vi "Diagnostics.Channel.Engine.vi"(8 "error in":errorcluster, 11 "State Variables":T1={"TCP Refs"={"Connection List"=refnum, "listener ID"=refnum}, "Stop"=refnum, "Top VI"=refnum, "Parameters"={"Properties"={"Name"="", "CAN"={"CAN Interface"=enum."CAN0", "Baud Rate"=0, "Diagnostic Protocol"=enum."GMLAN", "Transport Protocol"=enum."ISO TP - Normal Mode", "Transmit ID"=0, "Receive ID"=0, "Transmit Extension"=0, "Receive Extension"=0, "Receive UUDT ID"=0, "Enable Stream"=TRUE, "VW TP Channel ID"=0, "Security"={"Source DLL Path"=path "", "Security Level"=1, "Target DLL Path"=path ""}, "Fill Frame"=FALSE, "Fill Byte"=255, "Termination"=FALSE}, "986x"={"Enable"=FALSE, "RIO Device"=0, "Bitfile"=path ""}, "Reads"=[], "Frames Lookup"=variant, "Writes"=[], "DPIDs"=[], "DPID Lookup"=variant, "DTC descriptor"={"DTC Byte Length"=2, "Status Byte Length"=1, "Add Data Byte Length"=1, "Byte Order"=enum."Motorola"}, "Created DTCs"=0}, "ChanRefs"={"ToVS.Reads"={"Name"="", "Write to VS Engine FIFO"=refnum, "Pairs"={"Refs"=[], "Values"=[]}}, "ToVS.DTCs"={"Name"="", "Write to VS Engine FIFO"=refnum, "Pairs"={"Refs"=[], "Values"=[]}}, "ToVS.DTCCount"={"Name"="", "Write to VS Engine FIFO"=refnum, "Pairs"={"Refs"=[], "Values"=[]}}, "ToVS.Status"={"Name"="", "Write to VS Engine FIFO"=refnum, "Pairs"={"Refs"=[], "Values"=[]}}, "FromVS.Writes"={"Name"="", "Read from VS Engine FIFO"=refnum, "Pairs"={"Refs"=[], "Values"=[]}}, "Cmds"={"Name"="", "Write to VS Engine FIFO"=refnum, "Read from VS Engine FIFO"=refnum, "Pairs"={"Chan Refs"=[], "Prev. Values"=[]}}, "Triggers"={"Name"="", "Write to VS Engine FIFO"=refnum, "Read from VS Engine FIFO"=refnum, "Pairs"={"Chan Refs"=[], "Prev. Values"=[]}}}}, "ADCS Connection"={"Diag CAN Handle"=0, "Transport Protocol"=enum."ISO TP - Normal Mode", "Receive Address Extension"=0, "Transmit Address Extension"=0, "Receive CAN Id"=0, "Transmit CAN Id"=0, "Diag CAN Queue"=refnum, "Log Frames ?"=FALSE, "My TP Address"=0, "Other TP Address"=0, "T1"=0, "T2"=0, "T3"=0, "T4"=0, "Tx SN"=0, "Block Size"=0, "Rx SN"=0, "VW TP Initialized?"=FALSE, "Tx block no"=0, "baud rate"=0, "Interface"="", "Channel Diag CAN Handle"=0, "UDP Connection ID"=refnum, "TCP Connection ID"=refnum, "Target IP Addr"=0, "Source Address"=0, "Target Address"=0, "Send Header NACK?"=FALSE, "DLL Handle"=0, "NAD"=0, "Time Stamp read first"=0.0, "Time Stamp read last"=0.0, "Time Stamp write first"=0.0, "Time Stamp write last"=0.0, "Time Stamp write"=0.0, "Time Stamp read"=0.0}, "XNET References"={"Database"="", "GMLAN DPID Session"="", "Cluster"=""}, "BufferedCmds"=refnum, "XNETEngine (GMLAN)"=refnum} {"Parameters"."ChanRefs"."Triggers"."Pairs"."Chan Refs" format="%.0x"; "Parameters"."ChanRefs"."Cmds"."Pairs"."Chan Refs" format="%.0x"; "Parameters"."ChanRefs"."ToVS.Status"."Pairs"."Refs" format="%.0x"; "Parameters"."ChanRefs"."ToVS.DTCCount"."Pairs"."Refs" format="%.0x"; "Parameters"."ChanRefs"."ToVS.DTCs"."Pairs"."Refs" format="%.0x"; "Parameters"."ChanRefs"."ToVS.Reads"."Pairs"."Refs" format="%.0x"; "Parameters"."Properties"."Writes"."Signals"."Byte Order" items=["Little Endian", "Big Endian"]; "Parameters"."Properties"."Writes"."Signals"."Data Type" items=["Signed", "Unsigned", "IEEE Float"]; "Parameters"."Properties"."CAN"."Fill Byte" format="%.0x"; "Parameters"."Properties"."CAN"."VW TP Channel ID" format="%.0x"; "Parameters"."Properties"."CAN"."Receive UUDT ID" format="%.0x"; "Parameters"."Properties"."CAN"."Receive Extension" format="%.0x"; "Parameters"."Properties"."CAN"."Transmit Extension" format="%.0x"; "Parameters"."Properties"."CAN"."Receive ID" format="%.0x"; "Parameters"."Properties"."CAN"."Transmit ID" format="%.0x"; "Parameters"."Properties"."Reads"."Signals"."Byte Order" items=["Little Endian", "Big Endian"]; "Parameters"."Properties"."Reads"."Signals"."Data Type" items=["Signed", "Unsigned", "IEEE Float"]}) -> (0 "error out":errorcluster)   [LabVIEW 2015, in "Diagnostics Addon Engine.lvlib"]
uses:
  Diagnostics Addon Engine.lvlib
  Types/Diagnostics.State.ctl
  Types/TCP.Refs.ctl
  STM/STM Lookup Table Ref.ctl
  Stop FG/Stop Global Ref.ctl
  Types/Engine.State.ctl
  Shared/Types/SysDef.Compile.Properties.ctl
  Shared/Types/CAN.ctl
  Shared/Types/CAN.Interface.ctl
  Shared/Types/Protocol.ctl
  Shared/Types/Transport.ctl
  Shared/Types/Security.ctl
  Shared/Types/986x.ctl
  Shared/Types/Frame.Compile.ctl
  Shared/Types/Type.ctl
  Shared/Types/Signal.ctl
  Shared/Types/DPID.ctl
  Shared/Types/DPID.Rate.ctl
  Shared/Types/DTCDescriptor.ctl
  Types/Engine.Refs.ctl
  Inline Async API/Controls/Write To VS Engine.ctl
  <vilib>/NI Veristand/Custom Device API/Data Reference.ctl
  Inline Async API/Controls/Read From VS Engine.ctl
  <vilib>/NI Veristand/Custom Device API/Block Data Reference.ctl
  Inline Async API/Controls/ReadWrite Data.ctl
  <vilib>/Automotive Diagnostic Command Set/Diagnostic Transport.llb/Diag Reference.ctl
  <vilib>/Automotive Diagnostic Command Set/Diagnostic Transport.llb/Transport Protocol Selector.ctl
  <vilib>/Automotive Diagnostic Command Set/Diagnostic Transport.llb/Diag CAN Frame Log.ctl
  Types/XNET.Refs.ctl
  <vilib>/NI/AMC/Message Queue.ctl
  <vilib>/NI/AMC/Message.ctl
  <vilib>/NI/Tools/Keyed Array/KeyedArray.ctl
  Stop FG/Stop Global Commands.ctl
  Shared/Types/Command.ctl
  Shared/Types/Command.Memory.ctl
  Shared/Types/Command.ReadDTC.ctl
  Shared/Types/Command.ReadDTCbyDTCNumber.ctl
  Shared/Types/Command.Communication.ctl
  Shared/Types/Command.IO.ctl
  GMLAN/_SubVIs/ReadFailureRecordData_readFailureRecordParameters_failureRecordIdentifier.ctl
  Shared/Types/Command.PassThru.Channel.ctl
  <vilib>/NI/AMC/Update Message Routing Info.vi
  <vilib>/NI/AMC/Create Multiple Messages.vi
  <vilib>/NI/AMC/Create Single Message.vi
  <vilib>/NI/AMC/Send Message.vi
  Error Handling API/Error Handling API.lvlib
  Stop FG/Stop FG.lvlib
  Shared/Diagnostics Addon Shared.lvlib
  <vilib>/NI/AMC/AMC.lvlib
  GMLAN/GMLAN.lvlib
  <vilib>/NI Veristand/Custom Device API/Custom Device API.lvlib
  <vilib>/NI/Tools/Keyed Array/Tools_KeyedArray.lvlib
  <vilib>/addons/Automotive Diagnostic Command Set/NI_Automotive Diagnostic Command Set.lvlib
  Inline Async API/Inline Async API.lvlib
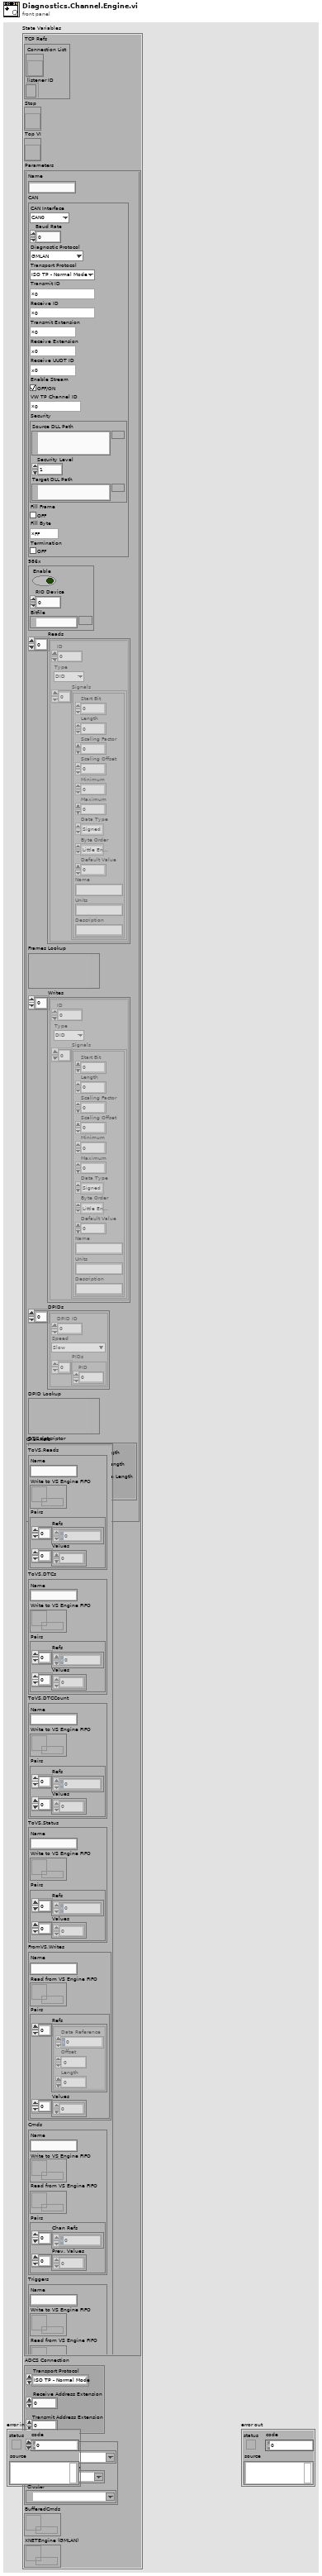
[diagram p1: front panel]
types:
  T1 = typedef "Diagnostics Addon Engine.lvlib/Diagnostics.State.ctl" = cluster{"TCP Refs":T2, "Stop":T4, "Top VI":refnum<vi>, "Parameters":T5, "ADCS Connection":T25, "XNET References":T27, "BufferedCmds":T28, "XNETEngine (GMLAN)":T28}
  T2 = typedef "Diagnostics Addon Engine.lvlib/TCP.Refs.ctl" = cluster{"Connection List":T3, "listener ID":refnum<k5>}
  T3 = typedef "Diagnostics Addon Engine.lvlib/STM Lookup Table Ref.ctl" = refnum<vi>
  T4 = typedef "Diagnostics Addon Engine.lvlib/Stop FG.lvlib/Stop Global Ref.ctl" = refnum<vi>
  T5 = typedef "Diagnostics Addon Engine.lvlib/Engine.State.ctl" = cluster{"Properties":T6, "ChanRefs":T19}
  T6 = typedef "Diagnostics Addon Shared.lvlib/SysDef.Compile.Properties.ctl" = cluster{"Name":string, "CAN":T7, "986x":T12, "Reads":T13[], "Frames Lookup":variant, "Writes":T13[], "DPIDs":T16[], "DPID Lookup":variant, "DTC descriptor":T18, "Created DTCs":u32}
  T7 = typedef "Diagnostics Addon Shared.lvlib/CAN.ctl" = cluster{"CAN Interface":T8, "Baud Rate":u32, "Diagnostic Protocol":T9, "Transport Protocol":T10, "Transmit ID":u32, "Receive ID":u32, "Transmit Extension":u8, "Receive Extension":u8, "Receive UUDT ID":u32, "Enable Stream":bool, "VW TP Channel ID":u32, "Security":T11, "Fill Frame":bool, "Fill Byte":u8, "Termination":bool}
  T8 = typedef "Diagnostics Addon Shared.lvlib/CAN.Interface.ctl" = enum16{"CAN0", "CAN1", "CAN2", "CAN3", "CAN4", "CAN5", "CAN6", "CAN7", "CAN8", "CAN9", "CAN10", "CAN11", "CAN12", "CAN13", "CAN14", "CAN15", "CAN16", "CAN17", "CAN18", "CAN19", "CAN20", "CAN21", "CAN22", "CAN23", "CAN24", "CAN25", "CAN26", "CAN27", "CAN28", "CAN29", "CAN30", "CAN31", "CAN32", "CAN33", "CAN34", "CAN35", "CAN36", "CAN37", "CAN38", "CAN39", "CAN40", "CAN41", "CAN42", "CAN43", "CAN44", "CAN45", "CAN46", "CAN47", "CAN48", "CAN49", "CAN50", "CAN51", "CAN52", "CAN53", "CAN54", "CAN55", "CAN56", "CAN57", "CAN58", "CAN59", "CAN60", "CAN61", "CAN62", "CAN63", "CAN 256 (Virtual)", "CAN 257 (Virtual)"}
  T9 = typedef "Diagnostics Addon Shared.lvlib/Protocol.ctl" = enum16{"GMLAN", "KWP-2000", "UDS", "User-Defined"}
  T10 = typedef "Diagnostics Addon Shared.lvlib/Transport.ctl" = enum16{"ISO TP - Normal Mode", "ISO TP - Mixed Mode", "VW TP 2.0", "Diagnostics on IP"}
  T11 = typedef "Diagnostics Addon Shared.lvlib/Security.ctl" = cluster{"Source DLL Path":path, "Security Level":u8, "Target DLL Path":path}
  T12 = typedef "Diagnostics Addon Shared.lvlib/986x.ctl" = cluster{"Enable":bool, "RIO Device":u16, "Bitfile":path}
  T13 = typedef "Diagnostics Addon Shared.lvlib/Frame.Compile.ctl" = cluster{"ID":u32, "Type":T14, "Signals":T15[]}
  T14 = typedef "Diagnostics Addon Shared.lvlib/Type.ctl" = enum16{"DID", "CDID", "PID", "CPID", "Read Memory", "Write Memory", "DTC Control", "IO Cmd", "IO Resp", "Routine Start Cmd", "Routine Start Resp", "Routine Request Cmd", "Routine Request Resp", "Routine Stop Cmd", "Routine Stop Resp", "UserDefined Cmd", "UserDefined Rsp"}
  T15 = typedef "Diagnostics Addon Shared.lvlib/Signal.ctl" = cluster{"Start Bit":u32, "Length":u32, "Scaling Factor":dbl, "Scaling Offset":dbl, "Minimum":dbl, "Maximum":dbl, "Data Type":u32, "Byte Order":u32, "Default Value":dbl, "Name":string, "Units":string, "Description":string}
  T16 = typedef "Diagnostics Addon Shared.lvlib/DPID.ctl" = cluster{"DPID ID":u8, "Speed":T17, "PIDs":u16[]}
  T17 = typedef "Diagnostics Addon Shared.lvlib/DPID.Rate.ctl" = enum16{"Slow", "Medium", "Fast"}
  T18 = typedef "Diagnostics Addon Shared.lvlib/DTCDescriptor.ctl" = cluster{"DTC Byte Length":i32, "Status Byte Length":i32, "Add Data Byte Length":i32, "Byte Order":enum16{"Motorola", "Intel"}}
  T19 = typedef "Diagnostics Addon Engine.lvlib/Engine.Refs.ctl" = cluster{"ToVS.Reads":T20, "ToVS.DTCs":T20, "ToVS.DTCCount":T20, "ToVS.Status":T20, "FromVS.Writes":T22, "Cmds":T24, "Triggers":T24}
  T20 = typedef "Diagnostics Addon Engine.lvlib/Inline Async API.lvlib/Write To VS Engine.ctl" = cluster{"Name":string, "Write to VS Engine FIFO":refnum<k33>, "Pairs":cluster{"Refs":T21[], "Values":dbl[]}}
  T21 = typedef "Custom Device API.lvlib/Data Reference.ctl" = i32
  T22 = typedef "Diagnostics Addon Engine.lvlib/Inline Async API.lvlib/Read From VS Engine.ctl" = cluster{"Name":string, "Read from VS Engine FIFO":refnum<k33>, "Pairs":cluster{"Refs":T23[], "Values":dbl[]}}
  T23 = typedef "Custom Device API.lvlib/Block Data Reference.ctl" = cluster{"Data Reference":T21, "Offset":u64, "Length":u64}
  T24 = typedef "Diagnostics Addon Engine.lvlib/Inline Async API.lvlib/ReadWrite Data.ctl" = cluster{"Name":string, "Write to VS Engine FIFO":refnum<k33>, "Read from VS Engine FIFO":refnum<k33>, "Pairs":cluster{"Chan Refs":T21[], "Prev. Values":dbl[]}}
  T25 = typedef "NI_Automotive Diagnostic Command Set.lvlib/Diag Reference.ctl" = cluster{"Diag CAN Handle":u32, "Transport Protocol":T26, "Receive Address Extension":u8, "Transmit Address Extension":u8, "Receive CAN Id":u32, "Transmit CAN Id":u32, "Diag CAN Queue":refnum<queue>, "Log Frames ?":bool, "My TP Address":u8, "Other TP Address":u8, "T1":u16, "T2":u16, "T3":u16, "T4":u16, "Tx SN":u8, "Block Size":u8, "Rx SN":u8, "VW TP Initialized?":bool, "Tx block no":u8, "baud rate":u32, "Interface":string, "Channel Diag CAN Handle":u32, "UDP Connection ID":refnum<k16>, "TCP Connection ID":refnum<k5>, "Target IP Addr":u32, "Source Address":u16, "Target Address":u16, "Send Header NACK?":bool, "DLL Handle":u32, "NAD":u8, "Time Stamp read first":dbl, "Time Stamp read last":dbl, "Time Stamp write first":dbl, "Time Stamp write last":dbl, "Time Stamp write":dbl, "Time Stamp read":dbl}
  T26 = typedef "NI_Automotive Diagnostic Command Set.lvlib/Transport Protocol Selector.ctl" = enum16{"ISO TP - Normal Mode", "ISO TP - Mixed Mode", "VW TP 2.0", "Diagnostics on IP", "ISO TP LIN"}
  T27 = typedef "Diagnostics Addon Engine.lvlib/XNET.Refs.ctl" = cluster{"Database":refnum<k21>, "GMLAN DPID Session":refnum<k21>, "Cluster":refnum<k21>}
  T28 = typedef "AMC.lvlib/Message Queue.ctl" = refnum<queue>
  T29 = typedef "Diagnostics Addon Engine.lvlib/Stop FG.lvlib/Stop Global Commands.ctl" = enum16{"Write", "Read", "Reset"}
  T30 = typedef "Diagnostics Addon Shared.lvlib/Command.ctl" = enum8{"None", "EnableDiagnosticSession", "DisableDiagnosticSession", "ReadDataIdentifiers", "ReadDataIdentifier", "WriteDataIndentifier", "ReadPIDsOnDemand", "ReadPIDOnDemand", "WriteCPID", "WriteMemory", "ReadMemory", "ReadDTCs", "ClearDTCs", "ControlDTC", "ForceTesterPresent", "DisableNormalCommunication", "ReturnToNormalMode", "InputOutputControl", "StartRoutine", "RequestRoutineStatus", "StopRoutine", "ECUReset", "UnlockECU", "ClearSuccessBit", "ConfigureandStartPIDs", "StopPIDs", "StartDTCs", "EnableChangeDTCCount", "DisableChangeDTCCount", "ReadFailureRecordParameters", "PassThru Channel Based", "EnableRepeatingTesterPresent", "DisableRepeatingTesterPresent"}
  T31 = typedef "Diagnostics Addon Shared.lvlib/Command.Memory.ctl" = cluster{"Address":u64, "Service Type":u32, "Address Length":u8, "Size Length":u8}
  T32 = typedef "Diagnostics Addon Shared.lvlib/Command.ReadDTC.ctl" = cluster{"Extension":u32, "Mask":u32, "Mode":u32}
  T33 = typedef "Diagnostics Addon Shared.lvlib/Command.ReadDTCbyDTCNumber.ctl" = cluster{"DTC":u16, "FailTypeByte":u8}
  T34 = typedef "Diagnostics Addon Shared.lvlib/Command.Communication.ctl" = cluster{"Type":u8, "CommType":u8}
  T35 = typedef "Diagnostics Addon Shared.lvlib/Command.IO.ctl" = cluster{"ID":u16, "Mode":u8}
  T36 = typedef "GMLAN.lvlib/ReadFailureRecordData_readFailureRecordParameters_failureRecordIdentifier.ctl" = cluster{"failureRecordNumber":u8, "DTC ID":u16, "DTCFailureType":u8}
  T37 = typedef "Diagnostics Addon Shared.lvlib/Command.PassThru.Channel.ctl" = cluster{"Service":u64, "Service Length":u8, "Data Length":u32, "Response Required":bool}
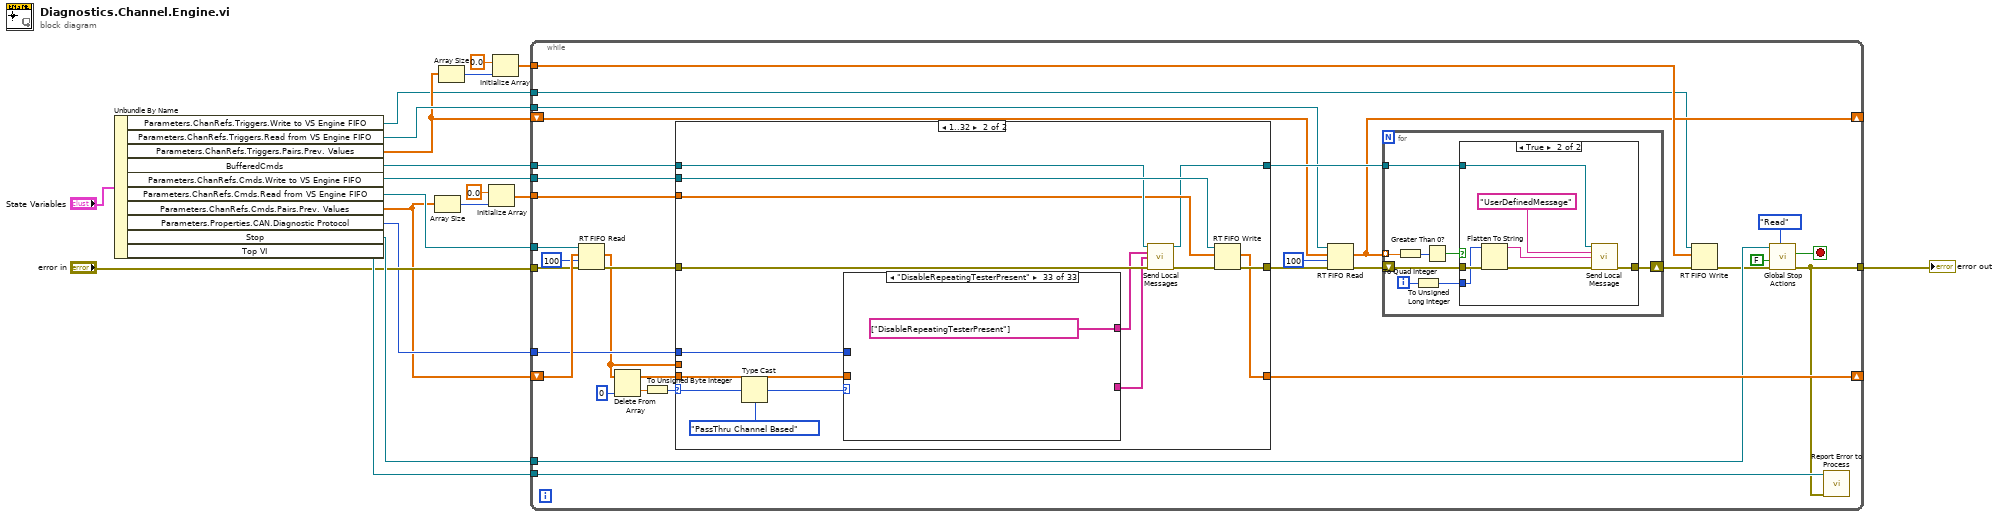
[diagram p0: block diagram]
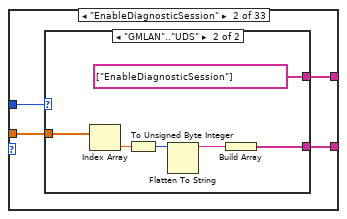
[diagram p5: hidden frame]
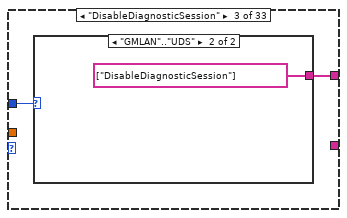
[diagram p7: hidden frame]
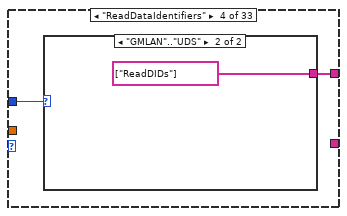
[diagram p9: hidden frame]
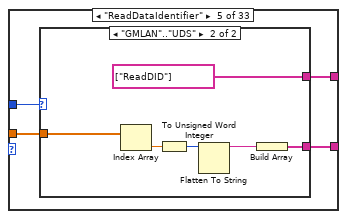
[diagram p11: hidden frame]
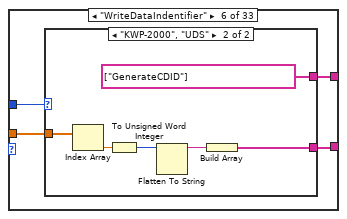
[diagram p13: hidden frame]
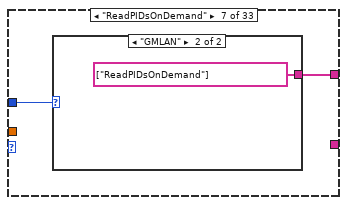
[diagram p15: hidden frame]
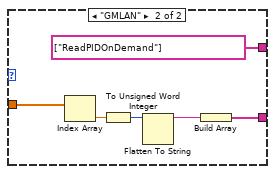
[diagram p18: hidden frame]
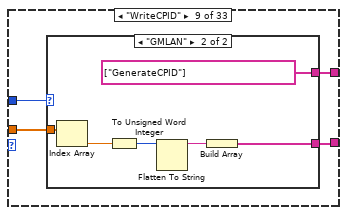
[diagram p19: hidden frame]
diagram:
  n1 = Unbundle By Name("State Variables") -> ("Parameters.ChanRefs.Triggers.Write to VS Engine FIFO"=w1:refnum<k33>, "Parameters.ChanRefs.Triggers.Read from VS Engine FIFO"=w3:refnum<k33>, "Parameters.ChanRefs.Triggers.Pairs.Prev. Values"=w2:dbl[], "BufferedCmds"=w12:T28, "Parameters.ChanRefs.Cmds.Write to VS Engine FIFO"=w13:refnum<k33>, "Parameters.ChanRefs.Cmds.Read from VS Engine FIFO"=w14:refnum<k33>, "Parameters.ChanRefs.Cmds.Pairs.Prev. Values"=w8:dbl[], "Parameters.Properties.CAN.Diagnostic Protocol"=w11:T9, "Stop"=w18:T4, "Top VI"=w17:refnum<vi>)
  n2 = Array Size(array=w8) -> (size(s)=w9:i32)
  n3 = Array Size(array=w2) -> (size(s)=w6:i32)
  n4 = Initialize Array(0.0 ("element"), w9) -> (w7:dbl[])
  n5 = Initialize Array(0.0 ("element"), w6) -> (w4:dbl[])
  n6 = while {
    tunnel: w14 -> [w46]
    shift-right: [w44] -> _
    shift-left: w8 -> [w45]
    tunnel: w18 -> [w40]
    tunnel: w17 -> [w39]
    tunnel: [w38] -> w16
    tunnel: "error in" -> [w36]
    tunnel: w13 -> [w35]
    tunnel: w12 -> [w34]
    tunnel: w11 -> [w33]
    tunnel: w7 -> [w30]
    tunnel: w4 -> [w25]
    tunnel: w3 -> [w23]
    shift-right: [w21] -> _
    shift-left: w2 -> [w22]
    tunnel: w1 -> [w20]
    stop <- w37 stop-if-true
    n7 = RT FIFO Read(0:w46, 1:w45, 2:100 ("timeout in ms (0)"), 3:w36) -> (9:w29:dbl[], 11:w51:errorcluster)  [unwired: 3 out]
    n8 = Delete From Array(array=w29, index=0) -> (deleted portion=w49:dbl, array with subset deleted=w47:dbl[])  [unwired: 1 in]
    n9 = To Unsigned Byte Integer(number=w49) -> (unsigned 8bit integer=w48:u8)
    n10 = case shown="1..32" w48 {
      selector: w48 -> [_ w73]
      tunnel: w51 -> [w70 w83]
      tunnel: w47 -> [_ w81]
      tunnel: [w69 w72] -> w44
      tunnel: [w70 w84] -> w31
      tunnel: w35 -> [_ w78]
      tunnel: w34 -> [w68 w75]
      tunnel: w33 -> [_ w74]
      tunnel: w30 -> [_ w72]
      tunnel: w29 -> [w69 _]
      tunnel: [w68 w71] -> w24
      frame 0, Default {
      }
      frame 1..32 {
        n11 = Type Cast(type=Command."PassThru Channel Based", x=w73) -> (*(type *) &x=w77:T30)
        n12 = case shown="\"DisableRepeatingTesterPresent\"" w77 {
          tunnel: w81 -> [_ w87 _ _ w103 w113 _ w126 w136 w145 w159 w174 w198 w208 w218 w229 _ w245 w259 w269 w279 w290 _ _ _ _ w310 w320 _ w336 w361 _ _]
          tunnel: [_ w88 w96 w99 w104 w114 w122 w127 w137 w147 w161 w175 w199 w209 w219 w230 w242 w247 w261 w271 w281 w291 w299 string[] ["ClearSuccessBit"] w303 w306 w311 w321 w330 w338 string[] ["ChannelPassThru"] string[] ["EnableRepeatingTesterPresent"] string[] ["DisableRepeatingTesterPresent"]] -> w80
          tunnel: [_ w86 _ _ w102 w112 _ w125 w135 w144 w158 w173 w197 w207 w217 w228 _ w244 w258 w268 w278 w289 _ _ _ _ w309 w319 w329 w337 w360 _ _] -> w79
          tunnel: w74 -> [_ w85 w95 w98 w101 w111 w121 w124 w134 w146 w160 w172 w196 w206 w216 w227 w241 w246 w260 w270 w280 w288 w298 _ w302 w305 w308 w318 w328 w335 _ _ _]
          frame "None" {
          }
          frame "EnableDiagnosticSession" {
            n13 = case shown="\"GMLAN\"..\"UDS\"" w85 {
              tunnel: [_ string[] ["EnableDiagnosticSession"]] -> w88
              tunnel: w87 -> [_ w90]
              tunnel: [_ w89] -> w86
              frame "User-Defined" {
              }
              frame "GMLAN".."UDS" {
                n14 = Index Array(array=w90) -> (element=w93:dbl)  [unwired: 1 in]
                n15 = To Unsigned Byte Integer(number=w93) -> (unsigned 8bit integer=w92:u8)
                n16 = Flatten To String(anything=w92) -> (data string=w91:string)  [unwired: 3 in, 2 out]
                n17 = Build Array(w91) -> (w89:string[])
              }
            }
          }
          frame "DisableDiagnosticSession" {
            n18 = case shown="\"GMLAN\"..\"UDS\"" w95 {
              tunnel: [_ string[] ["DisableDiagnosticSession"]] -> w96
              frame "User-Defined" {
              }
              frame "GMLAN".."UDS" {
              }
            }
          }
          frame "ReadDataIdentifiers" {
            n19 = case shown="\"GMLAN\"..\"UDS\"" w98 {
              tunnel: [_ string[] ["ReadDIDs"]] -> w99
              frame "User-Defined" {
              }
              frame "GMLAN".."UDS" {
              }
            }
          }
          frame "ReadDataIdentifier" {
            n20 = case shown="\"GMLAN\"..\"UDS\"" w101 {
              tunnel: [_ string[] ["ReadDID"]] -> w104
              tunnel: w103 -> [_ w106]
              tunnel: [_ w105] -> w102
              frame "User-Defined" {
              }
              frame "GMLAN".."UDS" {
                n21 = Index Array(array=w106) -> (element=w109:dbl)  [unwired: 1 in]
                n22 = To Unsigned Word Integer(number=w109) -> (unsigned 16bit integer=w108:u16)
                n23 = Flatten To String(anything=w108) -> (data string=w107:string)  [unwired: 3 in, 2 out]
                n24 = Build Array(w107) -> (w105:string[])
              }
            }
          }
          frame "WriteDataIndentifier" {
            n25 = case shown="\"KWP-2000\", \"UDS\"" w111 {
              tunnel: [_ string[] ["GenerateCDID"]] -> w114
              tunnel: w113 -> [_ w119]
              tunnel: [_ w118] -> w112
              frame "GMLAN", "User-Defined" {
              }
              frame "KWP-2000", "UDS" {
                n26 = Index Array(array=w119) -> (element=w117:dbl)  [unwired: 1 in]
                n27 = To Unsigned Word Integer(number=w117) -> (unsigned 16bit integer=w115:u16)
                n28 = Flatten To String(anything=w115) -> (data string=w116:string)  [unwired: 3 in, 2 out]
                n29 = Build Array(w116) -> (w118:string[])
              }
            }
          }
          frame "ReadPIDsOnDemand" {
            n30 = case shown="\"GMLAN\"" w121 {
              tunnel: [_ string[] ["ReadPIDsOnDemand"]] -> w122
              frame Default {
              }
              frame "GMLAN" {
              }
            }
          }
          frame "ReadPIDOnDemand" {
            n31 = case shown="Default" w124 {
              tunnel: [_ string[] ["ReadPIDOnDemand"]] -> w127
              tunnel: w126 -> [_ w129]
              tunnel: [_ w128] -> w125
              frame Default {
              }
              frame "GMLAN" {
                n32 = Index Array(array=w129) -> (element=w132:dbl)  [unwired: 1 in]
                n33 = To Unsigned Word Integer(number=w132) -> (unsigned 16bit integer=w131:u16)
                n34 = Flatten To String(anything=w131) -> (data string=w130:string)  [unwired: 3 in, 2 out]
                n35 = Build Array(w130) -> (w128:string[])
              }
            }
          }
          frame "WriteCPID" {
            n36 = case shown="\"GMLAN\"" w134 {
              tunnel: [_ string[] ["GenerateCPID"]] -> w137
              tunnel: w136 -> [_ w142]
              tunnel: [_ w141] -> w135
              frame Default {
              }
              frame "GMLAN" {
                n37 = Index Array(array=w142) -> (element=w140:dbl)  [unwired: 1 in]
                n38 = To Unsigned Word Integer(number=w140) -> (unsigned 16bit integer=w138:u16)
                n39 = Flatten To String(anything=w138) -> (data string=w139:string)  [unwired: 3 in, 2 out]
                n40 = Build Array(w139) -> (w141:string[])
              }
            }
          }
          frame "WriteMemory" {
            n41 = case shown="\"KWP-2000\", \"UDS\"" w146 {
              tunnel: [_ string[] ["WriteMemory"]] -> w147
              tunnel: w145 -> [_ w149]
              tunnel: [_ w156] -> w144
              frame "GMLAN", "User-Defined" {
              }
              frame "KWP-2000", "UDS" {
                n42 = Index Array(array=w149) -> (element #1=w153:dbl, element #2=w154:dbl, element #3=w152:dbl, element #4=w151:dbl)  [unwired: 4 in]
                n43 = Bundle By Name(cluster=T31 {"Address"=0, "Service Type"=0, "Address Length"=0, "Size Length"=0}, "Address"=w153, "Service Type"=w154, "Address Length"=w152, "Size Length"=w151) -> (w155:T31)
                n44 = Flatten To String(anything=w155) -> (data string=w150:string)  [unwired: 3 in, 2 out]
                n45 = Build Array(w150) -> (w156:string[])
              }
            }
          }
          frame "ReadMemory" {
            n46 = case shown="\"GMLAN\", \"User-Defined\"" w160 {
              tunnel: [_ string[] ["ReadMemory"]] -> w161
              tunnel: w159 -> [_ w170]
              tunnel: [_ w168] -> w158
              frame "GMLAN", "User-Defined" {
              }
              frame "KWP-2000", "UDS" {
                n47 = Index Array(array=w170) -> (element #1=w164:dbl, element #2=w165:dbl, element #3=w163:dbl, element #4=w162:dbl)  [unwired: 4 in]
                n48 = Bundle By Name(cluster=T31 {"Address"=0, "Service Type"=0, "Address Length"=0, "Size Length"=0}, "Address"=w164, "Service Type"=w165, "Address Length"=w163, "Size Length"=w162) -> (w166:T31)
                n49 = Flatten To String(anything=w166) -> (data string=w169:string)  [unwired: 3 in, 2 out]
                n50 = Build Array(w169) -> (w168:string[])
              }
            }
          }
          frame "ReadDTCs" {
            n51 = case shown="\"User-Defined\"" w172 {
              tunnel: [string[] ["ReadDTCs"] _ string[] ["ReadDTCByDTCNumber"]] -> w175
              tunnel: w174 -> [w183 _ w192]
              tunnel: [w181 _ w191] -> w173
              frame "KWP-2000", "UDS" {
                n52 = To Unsigned Long Integer(number=w183) -> (unsigned 32bit integer=w185:u32[])
                n53 = Index Array(array=w185) -> (element #1=w177:u32, element #2=w178:u32, element #3=w179:u32)  [unwired: 3 in]
                n54 = Bundle By Name(cluster=T32 {"Extension"=0, "Mask"=0, "Mode"=0}, "Extension"=w177, "Mask"=w178, "Mode"=w179) -> (w176:T32)
                n55 = Flatten To String(anything=w176) -> (data string=w184:string)  [unwired: 3 in, 2 out]
                n56 = Build Array(w184) -> (w181:string[])
              }
              frame "User-Defined" {
              }
              frame "GMLAN" {
                n57 = Index Array(array=w192) -> (element #1=w194:dbl, element #2=w190:dbl)  [unwired: 2 in]
                n58 = To Unsigned Word Integer(number=w194) -> (unsigned 16bit integer=w187:u16)
                n59 = To Unsigned Byte Integer(number=w190) -> (unsigned 8bit integer=w189:u8)
                n60 = Bundle By Name(cluster=T33 {"DTC"=0, "FailTypeByte"=0}, "DTC"=w187, "FailTypeByte"=w189) -> (w186:T33)
                n61 = Flatten To String(anything=w186) -> (data string=w193:string)  [unwired: 3 in, 2 out]
                n62 = Build Array(w193) -> (w191:string[])
              }
            }
          }
          frame "ClearDTCs" {
            n63 = case shown="\"User-Defined\"" w196 {
              tunnel: [_ string[] ["ClearDTCs"]] -> w199
              tunnel: w198 -> [_ w201]
              tunnel: [_ w200] -> w197
              frame "User-Defined" {
              }
              frame "GMLAN".."UDS" {
                n64 = Index Array(array=w201) -> (element=w204:dbl)  [unwired: 1 in]
                n65 = To Unsigned Long Integer(number=w204) -> (unsigned 32bit integer=w203:u32)
                n66 = Flatten To String(anything=w203) -> (data string=w202:string)  [unwired: 3 in, 2 out]
                n67 = Build Array(w202) -> (w200:string[])
              }
            }
          }
          frame "ControlDTC" {
            n68 = case shown="\"KWP-2000\", \"UDS\"" w206 {
              tunnel: [_ string[] ["ControlDTC"]] -> w209
              tunnel: w208 -> [_ w211]
              tunnel: [_ w210] -> w207
              frame "GMLAN", "User-Defined" {
              }
              frame "KWP-2000", "UDS" {
                n69 = Index Array(array=w211) -> (element=w214:dbl)  [unwired: 1 in]
                n70 = To Unsigned Long Integer(number=w214) -> (unsigned 32bit integer=w213:u32)
                n71 = Flatten To String(anything=w213) -> (data string=w212:string)  [unwired: 3 in, 2 out]
                n72 = Build Array(w212) -> (w210:string[])
              }
            }
          }
          frame "ForceTesterPresent" {
            n73 = case shown="\"User-Defined\"" w216 {
              tunnel: [_ string[] ["ForceTesterPresent"]] -> w219
              tunnel: w218 -> [_ w225]
              tunnel: [_ w224] -> w217
              frame "User-Defined" {
              }
              frame "GMLAN".."UDS" {
                n74 = Index Array(array=w225) -> (element=w223:dbl)  [unwired: 1 in]
                n75 = To Unsigned Byte Integer(number=w223) -> (unsigned 8bit integer=w220:u8)
                n76 = Number To Boolean Array(number=w220) -> (Boolean array=w221:bool[])
                n77 = Flatten To String(anything=w221) -> (data string=w222:string)  [unwired: 3 in, 2 out]
                n78 = Build Array(w222) -> (w224:string[])
              }
            }
          }
          frame "DisableNormalCommunication" {
            n79 = case shown="\"User-Defined\"" w227 {
              tunnel: [_ string[] ["DisableNormalCommunication"]] -> w230
              tunnel: w229 -> [_ w232]
              tunnel: [_ w231] -> w228
              frame "User-Defined" {
              }
              frame "GMLAN".."UDS" {
                n80 = Index Array(array=w232) -> (element #1=w237:dbl, element #2=w238:dbl)  [unwired: 2 in]
                n81 = To Unsigned Byte Integer(number=w238) -> (unsigned 8bit integer=w235:u8)
                n82 = To Unsigned Byte Integer(number=w237) -> (unsigned 8bit integer=w236:u8)
                n83 = Bundle By Name(cluster=T34 {"Type"=0, "CommType"=0} ("Cluster"), "Type"=w236, "CommType"=w235) -> (w234:T34)
                n84 = Flatten To String(anything=w234) -> (data string=w239:string)  [unwired: 3 in, 2 out]
                n85 = Build Array(w239) -> (w231:string[])
              }
            }
          }
          frame "ReturnToNormalMode" {
            n86 = case shown="\"User-Defined\"" w241 {
              tunnel: [_ string[] ["ReturnToNormalMode"]] -> w242
              frame "User-Defined" {
              }
              frame "GMLAN".."UDS" {
              }
            }
          }
          frame "InputOutputControl" {
            n87 = case shown="\"KWP-2000\", \"UDS\"" w246 {
              tunnel: [_ string[] ["InputOutputControl"]] -> w247
              tunnel: w245 -> [_ w255]
              tunnel: [_ w248] -> w244
              frame "GMLAN", "User-Defined" {
              }
              frame "KWP-2000", "UDS" {
                n88 = Index Array(array=w255) -> (element #1=w253:dbl, element #2=w254:dbl)  [unwired: 2 in]
                n89 = To Unsigned Byte Integer(number=w254) -> (unsigned 8bit integer=w250:u8)
                n90 = To Unsigned Word Integer(number=w253) -> (unsigned 16bit integer=w251:u16)
                n91 = Bundle By Name(cluster=T35 {"ID"=0, "Mode"=0}, "ID"=w251, "Mode"=w250) -> (w249:T35)
                n92 = Flatten To String(anything=w249) -> (data string=w256:string)  [unwired: 3 in, 2 out]
                n93 = Build Array(w256) -> (w248:string[])
              }
            }
          }
          frame "StartRoutine" {
            n94 = case shown="\"KWP-2000\", \"UDS\"" w260 {
              tunnel: [_ string[] ["StartRoutine"]] -> w261
              tunnel: w259 -> [_ w266]
              tunnel: [_ w262] -> w258
              frame "GMLAN", "User-Defined" {
              }
              frame "KWP-2000", "UDS" {
                n95 = Index Array(array=w266) -> (element=w265:dbl)  [unwired: 1 in]
                n96 = To Unsigned Word Integer(number=w265) -> (unsigned 16bit integer=w263:u16)
                n97 = Flatten To String(anything=w263) -> (data string=w264:string)  [unwired: 3 in, 2 out]
                n98 = Build Array(w264) -> (w262:string[])
              }
            }
          }
          frame "RequestRoutineStatus" {
            n99 = case shown="\"KWP-2000\", \"UDS\"" w270 {
              tunnel: [_ string[] ["RequestRoutineStatus"]] -> w271
              tunnel: w269 -> [_ w273]
              tunnel: [_ w272] -> w268
              frame "GMLAN", "User-Defined" {
              }
              frame "KWP-2000", "UDS" {
                n100 = Index Array(array=w273) -> (element=w276:dbl)  [unwired: 1 in]
                n101 = To Unsigned Word Integer(number=w276) -> (unsigned 16bit integer=w274:u16)
                n102 = Flatten To String(anything=w274) -> (data string=w275:string)  [unwired: 3 in, 2 out]
                n103 = Build Array(w275) -> (w272:string[])
              }
            }
          }
          frame "StopRoutine" {
            n104 = case shown="\"KWP-2000\", \"UDS\"" w280 {
              tunnel: [_ string[] ["StopRoutine"]] -> w281
              tunnel: w279 -> [_ w283]
              tunnel: [_ w282] -> w278
              frame "GMLAN", "User-Defined" {
              }
              frame "KWP-2000", "UDS" {
                n105 = Index Array(array=w283) -> (element=w286:dbl)  [unwired: 1 in]
                n106 = To Unsigned Word Integer(number=w286) -> (unsigned 16bit integer=w284:u16)
                n107 = Flatten To String(anything=w284) -> (data string=w285:string)  [unwired: 3 in, 2 out]
                n108 = Build Array(w285) -> (w282:string[])
              }
            }
          }
          frame "ECUReset" {
            n109 = case shown="\"KWP-2000\", \"UDS\"" w288 {
              tunnel: [_ string[] ["ECUReset"]] -> w291
              tunnel: w290 -> [_ w293]
              tunnel: [_ w292] -> w289
              frame "GMLAN", "User-Defined" {
              }
              frame "KWP-2000", "UDS" {
                n110 = Index Array(array=w293) -> (element=w296:dbl)  [unwired: 1 in]
                n111 = To Unsigned Byte Integer(number=w296) -> (unsigned 8bit integer=w295:u8)
                n112 = Flatten To String(anything=w295) -> (data string=w294:string)  [unwired: 3 in, 2 out]
                n113 = Build Array(w294) -> (w292:string[])
              }
            }
          }
          frame "UnlockECU" {
            n114 = case shown="\"GMLAN\"..\"UDS\"" w298 {
              tunnel: [_ string[] ["UnlockECU"]] -> w299
              frame "User-Defined" {
              }
              frame "GMLAN".."UDS" {
              }
            }
          }
          frame "ClearSuccessBit" {
          }
          frame "ConfigureandStartPIDs" {
            n115 = case shown="\"GMLAN\"" w302 {
              tunnel: [_ string[] ["ConfigurePIDs", "StartPIDs"]] -> w303
              frame Default {
              }
              frame "GMLAN" {
              }
            }
          }
          frame "StopPIDs" {
            n116 = case shown="\"GMLAN\"" w305 {
              tunnel: [_ string[] ["StopPIDs"]] -> w306
              frame Default {
              }
              frame "GMLAN" {
              }
            }
          }
          frame "StartDTCs" {
            n117 = case shown="\"GMLAN\"" w308 {
              tunnel: [string[] ["StartDTCs"] _] -> w311
              tunnel: w310 -> [w316 _]
              tunnel: [w312 _] -> w309
              frame "GMLAN" {
                n118 = Index Array(array=w316) -> (element=w315:dbl)  [unwired: 1 in]
                n119 = To Unsigned Byte Integer(number=w315) -> (unsigned 8bit integer=w314:u8)
                n120 = Flatten To String(anything=w314) -> (data string=w313:string)  [unwired: 3 in, 2 out]
                n121 = Build Array(w313) -> (w312:string[])
              }
              frame Default {
              }
            }
          }
          frame "EnableChangeDTCCount" {
            n122 = case shown="\"GMLAN\"" w318 {
              tunnel: [_ string[] ["EnableChangeDTCCount"]] -> w321
              tunnel: w320 -> [_ w326]
              tunnel: [_ w322] -> w319
              frame Default {
              }
              frame "GMLAN" {
                n123 = Index Array(array=w326) -> (element=w325:dbl)  [unwired: 1 in]
                n124 = To Unsigned Byte Integer(number=w325) -> (unsigned 8bit integer=w324:u8)
                n125 = Flatten To String(anything=w324) -> (data string=w323:string)  [unwired: 3 in, 2 out]
                n126 = Build Array(w323) -> (w322:string[])
              }
            }
          }
          frame "DisableChangeDTCCount" {
            n127 = case shown="\"GMLAN\"" w328 {
              tunnel: [_ string[] ["DisableChangeDTCCount"]] -> w330
              tunnel: [_ w332] -> w329
              frame Default {
              }
              frame "GMLAN" {
                n128 = Flatten To String(anything=u8 0 ("number")) -> (data string=w333:string)  [unwired: 3 in, 2 out]
                n129 = Build Array(w333) -> (w332:string[])
              }
            }
          }
          frame "ReadFailureRecordParameters" {
            n130 = case shown="\"GMLAN\"" w335 {
              tunnel: [_ string[] ["ReadFailureRecordParameters"]] -> w338
              tunnel: [_ w344] -> w337
              tunnel: w336 -> [_ w343]
              frame Default {
              }
              frame "GMLAN" {
                n131 = Index Array(array=w343) -> (element #1=w349:dbl, element #2=w347:dbl, element #3=w339:dbl)  [unwired: 3 in]
                n132 = To Unsigned Word Integer(number=w349) -> (unsigned 16bit integer=w346:u16)
                n133 = To Unsigned Byte Integer(number=w347) -> (unsigned 8bit integer=w341:u8)
                n134 = To Unsigned Byte Integer(number=w339) -> (unsigned 8bit integer=w340:u8)
                n135 = Bundle By Name(cluster=T36 {"failureRecordNumber"=0, "DTC ID"=0, "DTCFailureType"=0} ("failureRecordIdentifier"), "DTC ID"=w346, "DTCFailureType"=w341, "failureRecordNumber"=w340) -> (w345:T36)
                n136 = Flatten To String(anything=w345) -> (data string=w348:string)  [unwired: 3 in, 2 out]
                n137 = Build Array(w348) -> (w344:string[])
              }
            }
          }
          frame "PassThru Channel Based" {
            n138 = Index Array(array=w361) -> (element #1=w357:dbl, element #2=w358:dbl, element #3=w356:dbl, element #4=w353:dbl)  [unwired: 4 in]
            n139 = To Unsigned Byte Integer(number=w353) -> (unsigned 8bit integer=w352:u8)
            n140 = Greater Than 0?(x=w352) -> (x > 0?=w351:bool)
            n141 = Bundle By Name(cluster=T37 {"Service"=0, "Service Length"=0, "Data Length"=0, "Response Required"=FALSE}, "Service"=w357, "Service Length"=w358, "Data Length"=w356, "Response Required"=w351) -> (w359:T37)
            n142 = Flatten To String(anything=w359) -> (data string=w355:string)  [unwired: 3 in, 2 out]
            n143 = Build Array(w355) -> (w360:string[])
          }
          frame "EnableRepeatingTesterPresent" {
          }
          frame "DisableRepeatingTesterPresent" {
          }
        }
        n144 = call <vilib>:"Send Local Messages.vi"("message queue in"=w75, "message names"=w80, "message values"=w79, "error in"=w83) -> ("message queue out"=w71:T28, "error out"=w82:errorcluster)  [unwired: 9 in, 1 out]
        n145 = RT FIFO Write(0:w78, 1:w72, 3:w82) -> (11:w84:errorcluster)  [unwired: 2 in, 3 out]
      }
    }
    n146 = RT FIFO Read(0:w23, 1:w22, 2:100 ("timeout in ms (0)"), 3:w31) -> (9:w21:dbl[], 11:w28:errorcluster)  [unwired: 3 out]
    n147 = for {
      shift-right: [w55] -> w27
      shift-left: w28 -> [w56]
      tunnel: w21 -> [w59] mode=indexing
      tunnel: w24 -> [w53]
      i -> [w54]
      n148 = To Quad Integer(1:w59) -> (0:w58:i64)
      n149 = To Unsigned Long Integer(number=w54) -> (unsigned 32bit integer=w52:u32)
      n150 = Greater Than 0?(x=w58) -> (x > 0?=w57:bool)
      n151 = case shown="True" w57 {
        tunnel: w56 -> [w60 w67]
        tunnel: [w60 w66] -> w55
        tunnel: w52 -> [_ w64]
        tunnel: w53 -> [_ w62]
        frame False {
        }
        frame True {
          n152 = Flatten To String(anything=w64, error in (no error)=w67) -> (data string=w63:string, error out=w65:errorcluster)  [unwired: 2 in, 1 out]
          n153 = call <vilib>:"Send Local Message.vi"("message queue in"=w62, "message name"="UserDefinedMessage", "message value"=w63, "error in"=w65) -> ("error out"=w66:errorcluster)  [unwired: 9 in, 2 out]
        }
      }
    }
    n154 = RT FIFO Write(0:w20, 1:w25, 3:w27) -> (11:w26:errorcluster)  [unwired: 2 in, 3 out]
    n155 = call "Global Stop Actions.vi"("Command"=Stop_Global_Commands."Read", "error in (no error)"=w26, "Stop on Error?"=FALSE, "vi reference"=w40) -> ("error out"=w38:errorcluster, "Latched Stop"=w37:bool)  [unwired: 5 in, 1 out]
    n156 = call "Report Error to Process.vi"("Error"=w38, "This VI"=w39) -> ()  [unwired: 10 in]
  }
  "error out" <- w16
